vi "TextTo1dArray.vi"(0 "input string":string, 11 "error in":errorcluster) -> (4 "Array":string[](array[string]), 15 "error out":errorcluster)   [LabVIEW 2023, in "Unit Testing CA1.lvlib"]
uses:
  Unit Testing CA1.lvlib
  <vilib>/Utility/error.llb/Trim Whitespace One-Sided.vi
  <vilib>/regexp/Match Regular Expression.xnode
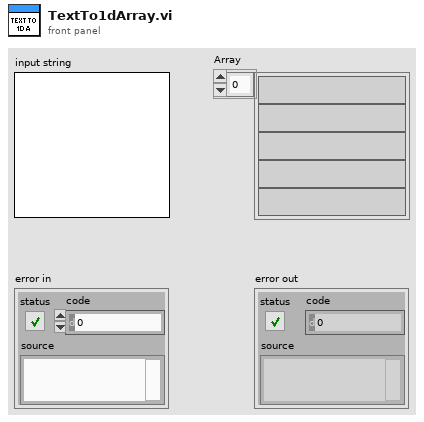
[diagram p1: front panel]
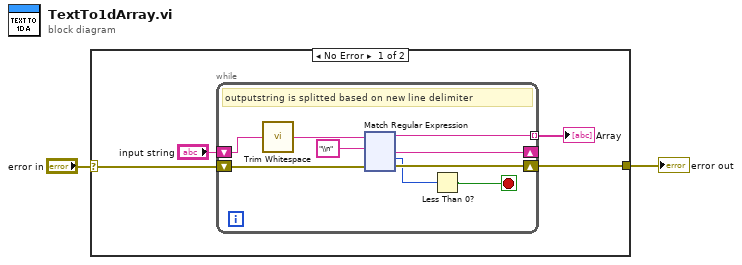
[diagram p0: block diagram]
diagram:
  n1 = case shown="No Error" "error in" {
    selector: "error in" -> [w4 w133]
    tunnel: [w5 w133] -> w2
    frame No Error {
      n2 = while {
        shift-right: [w10] -> _
        shift-left: "input string" -> [w15]
        tunnel: [w11] -> w3 mode=indexing
        shift-right: [w13] -> w5
        shift-left: w4 -> [w12]
        stop <- w8 stop-if-true
        # "outputstring is splitted based on new line delimiter"
        n3 = call <vilib>:"Trim Whitespace.vi"("string"=w15) -> ("trimmed string"=w7:string)  [unwired: 1 in]
        n4 = xnode "Match Regular Expression"("input string"=w7, "regular expression"="\\n", "error in"=w12) -> ("before match"=w11:string, "after match"=w10:string, "offset past match"=w9:i32, "error out"=w13:errorcluster)  [unwired: 3 in, 1 out]
        n5 = Less Than 0?(x=w9) -> (x < 0?=w8:bool)
      }
      "Array" <- w3
    }
    frame Error {
    }
  }
  "error out" <- w2
